vi "Parse Labels.vi"(8 "error in":errorcluster, 10 "Mod8/Rx0":u32, 11 "Arinc In":sgl[](array[numeric])) -> (0 "error out":errorcluster, 3 "Arinc Out":sgl[](array[numeric]))   [LabVIEW 2018, in "ARINC.lvlib"]
uses:
  ARINC.lvlib
panel:
  out "Data":u32
  out "Label":string
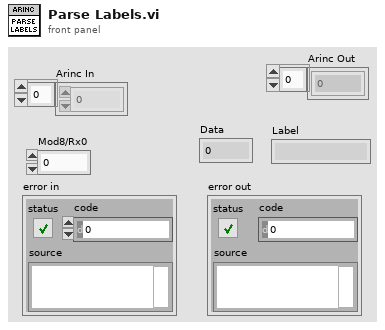
[diagram p1: front panel]
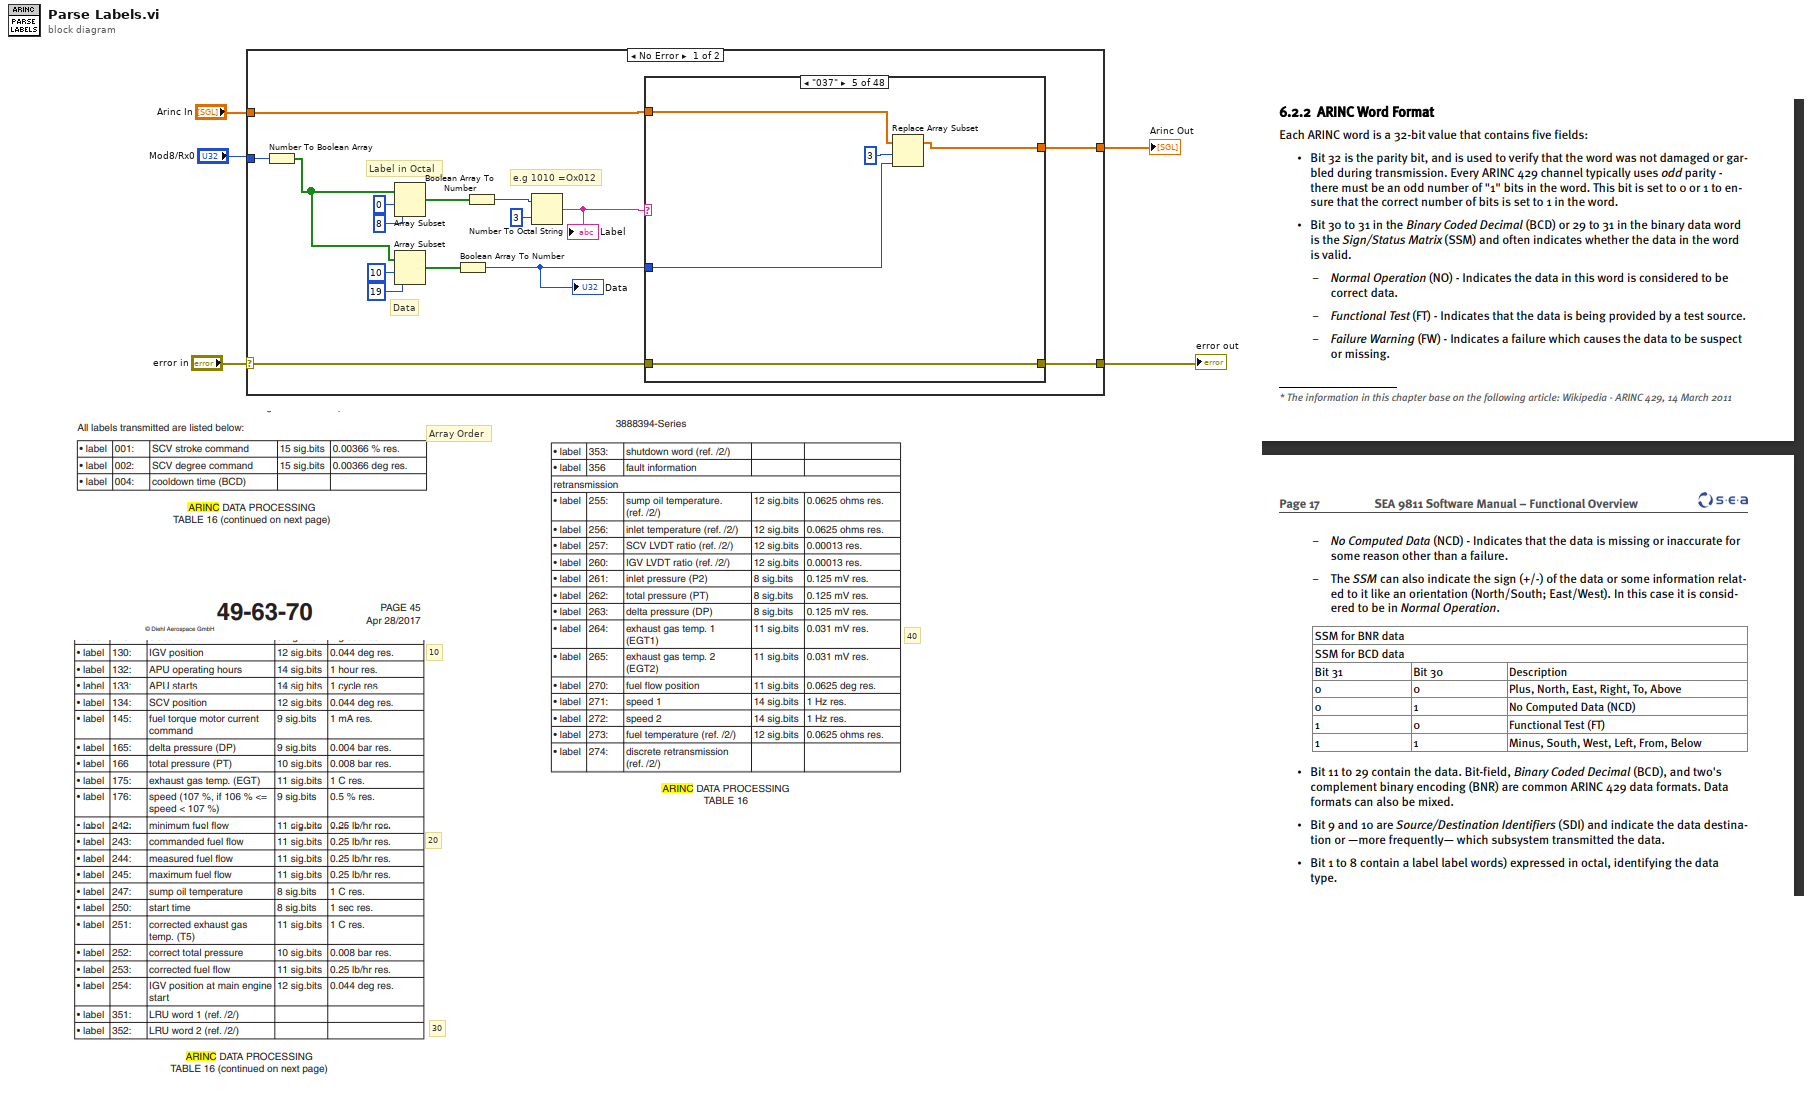
[diagram p0: block diagram]
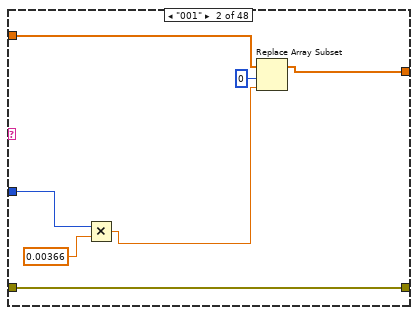
[diagram p3: hidden frame]
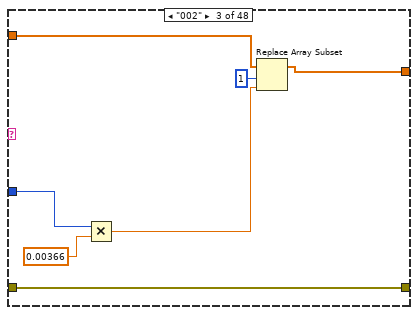
[diagram p4: hidden frame]
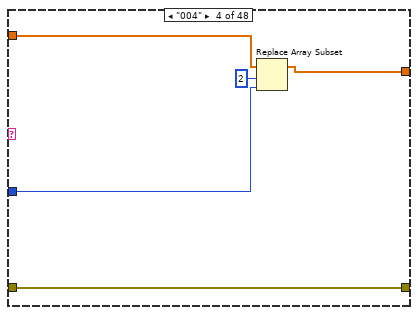
[diagram p5: hidden frame]
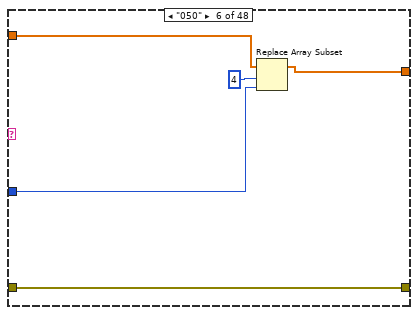
[diagram p6: hidden frame]
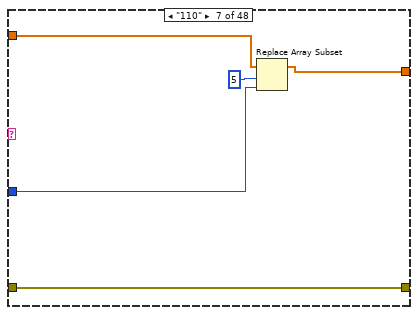
[diagram p7: hidden frame]
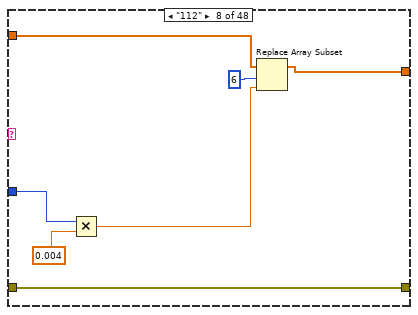
[diagram p8: hidden frame]
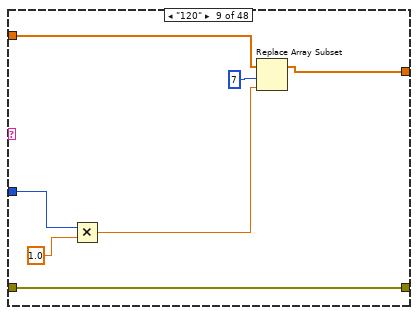
[diagram p9: hidden frame]
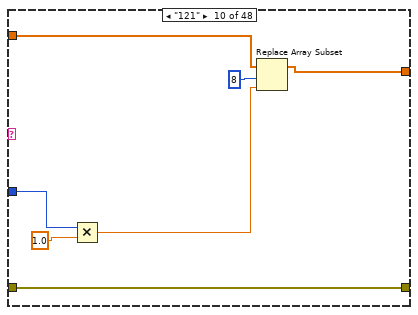
[diagram p10: hidden frame]
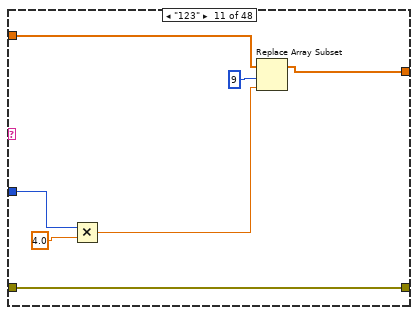
[diagram p11: hidden frame]
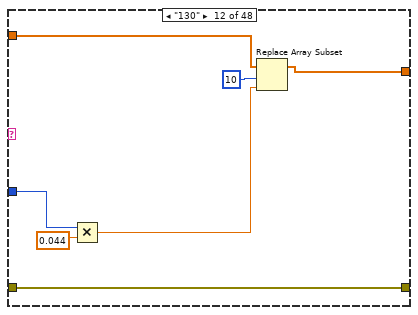
[diagram p12: hidden frame]
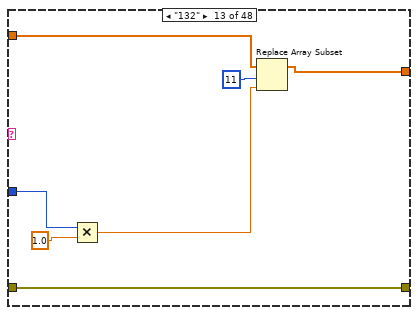
[diagram p13: hidden frame]
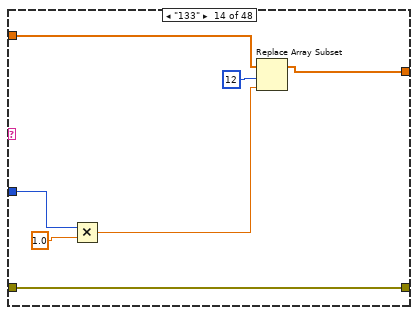
[diagram p14: hidden frame]
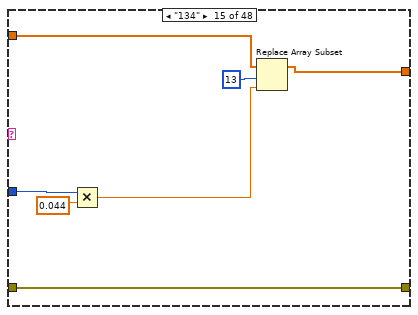
[diagram p15: hidden frame]
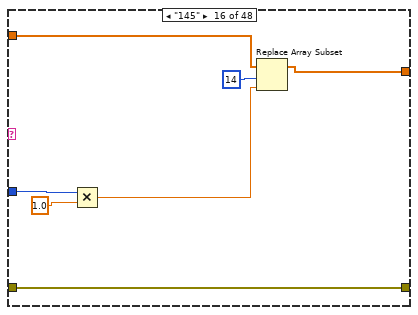
[diagram p16: hidden frame]
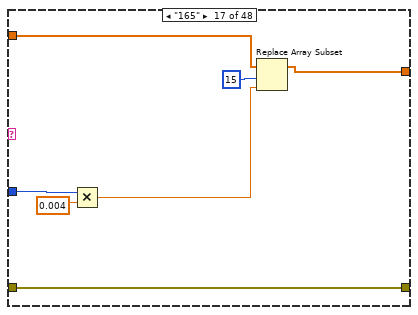
[diagram p17: hidden frame]
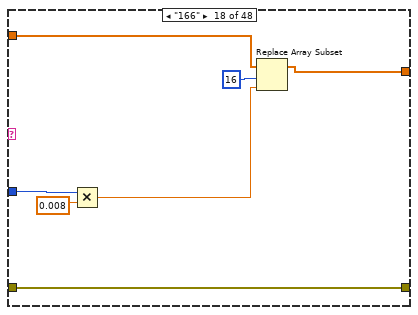
[diagram p18: hidden frame]
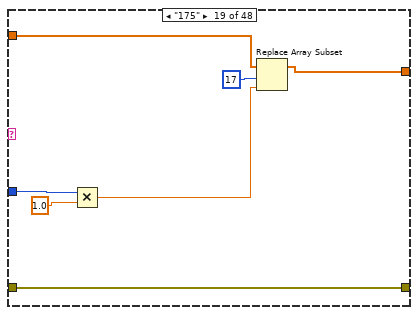
[diagram p19: hidden frame]
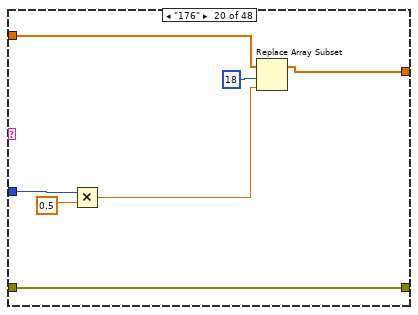
[diagram p20: hidden frame]
diagram:
  # "40"
  # "30"
  # "20"
  # "10"
  # "Array Order"
  n1 = case shown="No Error" "error in" {
    selector: "error in" -> [w7 w346]
    tunnel: "Mod8/Rx0" -> [w21 _]
    tunnel: [w6 w346] -> w5
    tunnel: "Arinc In" -> [w10 w345]
    tunnel: [w8 w345] -> w1
    frame No Error {
      # "e.g 1010 =Ox012"
      # "Data"
      # "Label in Octal"
      n2 = Number To Boolean Array(number=w21) -> (Boolean array=w16:bool[])
      n3 = Array Subset(array=w16, index=0, length=8) -> (w15:bool[])
      n4 = Array Subset(array=w16, index=10, length=19) -> (w14:bool[])
      n5 = Boolean Array To Number(Boolean array=w14) -> (number=w9:u32)
      "Data" <- w9
      n6 = Boolean Array To Number(Boolean array=w15) -> (number=w13:u32)
      n7 = Number To Octal String(1:i16 3 ("width (-)"), 2:w13) -> (0:w12:string)
      "Label" <- w12
      n8 = case shown="\"037\"" w12 {
        tunnel: w10 -> [w23 w30 w37 w42 w47 w52 w57 w64 w71 w78 w85 w92 w99 w106 w113 w120 w127 w134 w141 w148 w155 w162 w169 w176 w183 w190 w197 w204 w211 w218 w225 w232 w239 w246 w253 w260 w267 w274 w281 w288 w295 w302 w309 w316 w323 w330 w337 w344]
        tunnel: w9 -> [_ w28 w35 w40 w45 w50 w55 w62 w69 w76 w83 w90 w97 w104 w111 w118 w125 w132 w139 w146 w153 w160 w167 w174 w181 w188 w195 w202 w209 w216 w223 w230 w237 w244 w251 w258 w265 w272 w279 w286 w293 w300 w307 w314 w321 w328 w335 w342]
        tunnel: [w23 w26 w32 w39 w44 w49 w54 w60 w67 w74 w81 w88 w95 w102 w109 w116 w123 w130 w137 w144 w151 w158 w165 w172 w179 w186 w193 w200 w207 w214 w221 w228 w235 w242 w249 w256 w263 w270 w277 w284 w291 w298 w305 w312 w319 w326 w333 w339] -> w8
        tunnel: w7 -> [w22 w25 w31 w38 w43 w48 w53 w58 w65 w72 w79 w86 w93 w100 w107 w114 w121 w128 w135 w142 w149 w156 w163 w170 w177 w184 w191 w198 w205 w212 w219 w226 w233 w240 w247 w254 w261 w268 w275 w282 w289 w296 w303 w310 w317 w324 w331 w338]
        tunnel: [w22 w25 w31 w38 w43 w48 w53 w58 w65 w72 w79 w86 w93 w100 w107 w114 w121 w128 w135 w142 w149 w156 w163 w170 w177 w184 w191 w198 w205 w212 w219 w226 w233 w240 w247 w254 w261 w268 w275 w282 w289 w296 w303 w310 w317 w324 w331 w338] -> w6
        frame Default {
        }
        frame "001" {
          n9 = Multiply(x=w28, y=0.00366) -> (x*y=w24:dbl)
          n10 = Replace Array Subset(array=w30, new element=w24, index=0) -> (w26:sgl[])
        }
        frame "002" {
          n11 = Multiply(x=w35, y=0.00366) -> (x*y=w33:dbl)
          n12 = Replace Array Subset(array=w37, new element=w33, index=1) -> (w32:sgl[])
        }
        frame "004" {
          n13 = Replace Array Subset(array=w42, new element=w40, index=2) -> (w39:sgl[])
        }
        frame "037" {
          n14 = Replace Array Subset(array=w47, new element=w45, index=3) -> (w44:sgl[])
        }
        frame "050" {
          n15 = Replace Array Subset(array=w52, new element=w50, index=4) -> (w49:sgl[])
        }
        frame "110" {
          n16 = Replace Array Subset(array=w57, new element=w55, index=5) -> (w54:sgl[])
        }
        frame "112" {
          n17 = Multiply(x=w62, y=0.004) -> (x*y=w61:dbl)
          n18 = Replace Array Subset(array=w64, new element=w61, index=6) -> (w60:sgl[])
        }
        frame "120" {
          n19 = Multiply(x=w69, y=1.0) -> (x*y=w68:dbl)
          n20 = Replace Array Subset(array=w71, new element=w68, index=7) -> (w67:sgl[])
        }
        frame "121" {
          n21 = Multiply(x=w76, y=1.0) -> (x*y=w75:dbl)
          n22 = Replace Array Subset(array=w78, new element=w75, index=8) -> (w74:sgl[])
        }
        frame "123" {
          n23 = Multiply(x=w83, y=4.0) -> (x*y=w82:dbl)
          n24 = Replace Array Subset(array=w85, new element=w82, index=9) -> (w81:sgl[])
        }
        frame "130" {
          n25 = Multiply(x=w90, y=0.044) -> (x*y=w89:dbl)
          n26 = Replace Array Subset(array=w92, new element=w89, index=10) -> (w88:sgl[])
        }
        frame "132" {
          n27 = Multiply(x=w97, y=1.0) -> (x*y=w96:dbl)
          n28 = Replace Array Subset(array=w99, new element=w96, index=11) -> (w95:sgl[])
        }
        frame "133" {
          n29 = Multiply(x=w104, y=1.0) -> (x*y=w103:dbl)
          n30 = Replace Array Subset(array=w106, new element=w103, index=12) -> (w102:sgl[])
        }
        frame "134" {
          n31 = Multiply(x=w111, y=0.044) -> (x*y=w110:dbl)
          n32 = Replace Array Subset(array=w113, new element=w110, index=13) -> (w109:sgl[])
        }
        frame "145" {
          n33 = Multiply(x=w118, y=1.0) -> (x*y=w117:dbl)
          n34 = Replace Array Subset(array=w120, new element=w117, index=14) -> (w116:sgl[])
        }
        frame "165" {
          n35 = Multiply(x=w125, y=0.004) -> (x*y=w124:dbl)
          n36 = Replace Array Subset(array=w127, new element=w124, index=15) -> (w123:sgl[])
        }
        frame "166" {
          n37 = Multiply(x=w132, y=0.008) -> (x*y=w131:dbl)
          n38 = Replace Array Subset(array=w134, new element=w131, index=16) -> (w130:sgl[])
        }
        frame "175" {
          n39 = Multiply(x=w139, y=1.0) -> (x*y=w138:dbl)
          n40 = Replace Array Subset(array=w141, new element=w138, index=17) -> (w137:sgl[])
        }
        frame "176" {
          n41 = Multiply(x=w146, y=0.5) -> (x*y=w145:dbl)
          n42 = Replace Array Subset(array=w148, new element=w145, index=18) -> (w144:sgl[])
        }
        frame "242" {
          n43 = Multiply(x=w153, y=0.25) -> (x*y=w152:dbl)
          n44 = Replace Array Subset(array=w155, new element=w152, index=19) -> (w151:sgl[])
        }
        frame "243" {
          n45 = Multiply(x=w160, y=0.25) -> (x*y=w159:dbl)
          n46 = Replace Array Subset(array=w162, new element=w159, index=20) -> (w158:sgl[])
        }
        frame "244" {
          n47 = Multiply(x=w167, y=0.25) -> (x*y=w166:dbl)
          n48 = Replace Array Subset(array=w169, new element=w166, index=21) -> (w165:sgl[])
        }
        frame "245" {
          n49 = Multiply(x=w174, y=0.25) -> (x*y=w173:dbl)
          n50 = Replace Array Subset(array=w176, new element=w173, index=22) -> (w172:sgl[])
        }
        frame "247" {
          n51 = Multiply(x=w181, y=1.0) -> (x*y=w180:dbl)
          n52 = Replace Array Subset(array=w183, new element=w180, index=23) -> (w179:sgl[])
        }
        frame "250" {
          n53 = Multiply(x=w188, y=1.0) -> (x*y=w187:dbl)
          n54 = Replace Array Subset(array=w190, new element=w187, index=24) -> (w186:sgl[])
        }
        frame "251" {
          n55 = Multiply(x=w195, y=1.0) -> (x*y=w194:dbl)
          n56 = Replace Array Subset(array=w197, new element=w194, index=25) -> (w193:sgl[])
        }
        frame "252" {
          n57 = Multiply(x=w202, y=0.008) -> (x*y=w201:dbl)
          n58 = Replace Array Subset(array=w204, new element=w201, index=26) -> (w200:sgl[])
        }
        frame "253" {
          n59 = Multiply(x=w209, y=0.25) -> (x*y=w208:dbl)
          n60 = Replace Array Subset(array=w211, new element=w208, index=27) -> (w207:sgl[])
        }
        frame "254" {
          n61 = Multiply(x=w216, y=0.044) -> (x*y=w215:dbl)
          n62 = Replace Array Subset(array=w218, new element=w215, index=28) -> (w214:sgl[])
        }
        frame "351" {
          n63 = Multiply(x=w223, y=1.0) -> (x*y=w222:dbl)
          n64 = Replace Array Subset(array=w225, new element=w222, index=29) -> (w221:sgl[])
        }
        frame "352" {
          n65 = Multiply(x=w230, y=1.0) -> (x*y=w229:dbl)
          n66 = Replace Array Subset(array=w232, new element=w229, index=30) -> (w228:sgl[])
        }
        frame "353" {
          n67 = Multiply(x=w237, y=1.0) -> (x*y=w236:dbl)
          n68 = Replace Array Subset(array=w239, new element=w236, index=31) -> (w235:sgl[])
        }
        frame "356" {
          n69 = Multiply(x=w244, y=1.0) -> (x*y=w243:dbl)
          n70 = Replace Array Subset(array=w246, new element=w243, index=32) -> (w242:sgl[])
        }
        frame "255" {
          n71 = Multiply(x=w251, y=0.0625) -> (x*y=w250:dbl)
          n72 = Replace Array Subset(array=w253, new element=w250, index=33) -> (w249:sgl[])
        }
        frame "256" {
          n73 = Multiply(x=w258, y=0.0625) -> (x*y=w257:dbl)
          n74 = Replace Array Subset(array=w260, new element=w257, index=34) -> (w256:sgl[])
        }
        frame "257" {
          n75 = Multiply(x=w265, y=0.00013) -> (x*y=w264:dbl)
          n76 = Replace Array Subset(array=w267, new element=w264, index=35) -> (w263:sgl[])
        }
        frame "260" {
          n77 = Multiply(x=w272, y=0.00013) -> (x*y=w271:dbl)
          n78 = Replace Array Subset(array=w274, new element=w271, index=36) -> (w270:sgl[])
        }
        frame "261" {
          n79 = Multiply(x=w279, y=0.125) -> (x*y=w278:dbl)
          n80 = Replace Array Subset(array=w281, new element=w278, index=37) -> (w277:sgl[])
        }
        frame "262" {
          n81 = Multiply(x=w286, y=0.125) -> (x*y=w285:dbl)
          n82 = Replace Array Subset(array=w288, new element=w285, index=38) -> (w284:sgl[])
        }
        frame "263" {
          n83 = Multiply(x=w293, y=0.125) -> (x*y=w292:dbl)
          n84 = Replace Array Subset(array=w295, new element=w292, index=39) -> (w291:sgl[])
        }
        frame "264" {
          n85 = Multiply(x=w300, y=0.031) -> (x*y=w299:dbl)
          n86 = Replace Array Subset(array=w302, new element=w299, index=40) -> (w298:sgl[])
        }
        frame "265" {
          n87 = Multiply(x=w307, y=0.031) -> (x*y=w306:dbl)
          n88 = Replace Array Subset(array=w309, new element=w306, index=41) -> (w305:sgl[])
        }
        frame "270" {
          n89 = Multiply(x=w314, y=0.0625) -> (x*y=w313:dbl)
          n90 = Replace Array Subset(array=w316, new element=w313, index=42) -> (w312:sgl[])
        }
        frame "271" {
          n91 = Multiply(x=w321, y=1.0) -> (x*y=w320:dbl)
          n92 = Replace Array Subset(array=w323, new element=w320, index=43) -> (w319:sgl[])
        }
        frame "272" {
          n93 = Multiply(x=w328, y=1.0) -> (x*y=w327:dbl)
          n94 = Replace Array Subset(array=w330, new element=w327, index=44) -> (w326:sgl[])
        }
        frame "273" {
          n95 = Multiply(x=w335, y=0.0625) -> (x*y=w334:dbl)
          n96 = Replace Array Subset(array=w337, new element=w334, index=45) -> (w333:sgl[])
        }
        frame "274" {
          n97 = Multiply(x=w342, y=1.0) -> (x*y=w341:dbl)
          n98 = Replace Array Subset(array=w344, new element=w341, index=46) -> (w339:sgl[])
        }
      }
    }
    frame Error {
    }
  }
  "error out" <- w5
  "Arinc Out" <- w1
